vi "EMD8216 socket port change.vi"(10 "Remote_port":u16, 11 "CardID":u32) -> (3 "error_code":u32)   [LabVIEW 2009, in "EMD8216_64.lvlib"]
doc: "EMD8216Status EMD8216_socket_port_change(u32 CardID,u16 Remote_port);"
uses:
  EMD8216_64.lvlib
  <userlib>/EMD8216_64/EMD8216_64.dll
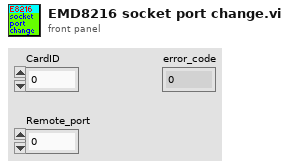
[diagram p1: front panel]
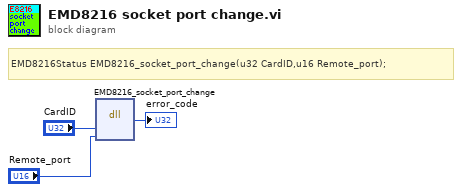
[diagram p0: block diagram]
diagram:
  # "EMD8216Status EMD8216_socket_port_change(u32 CardID,u16 Remote_port);"
  n1 = dll-call lib="C:/Program Files/National Instruments/LabVIEW 2017/user.lib/EMD8216_64/EMD8216_64.*" fn="EMD8216_socket_port_change"("CardID"="CardID", "Remote_port"="Remote_port") -> (→"error_code":u32)  [unwired: 5 in, 2 out]
